vi "Write Interlock.vi"(8 "error in (no error)":errorcluster, 10 "Interlock":bool, 11 "Oven in":refnum<class "Oven.lvclass">) -> (0 "error out":errorcluster, 3 "Oven out":refnum<class "Oven.lvclass">)   [LabVIEW 2018, in "Oven.lvlib" / "Oven.lvclass"]
uses:
  Oven.lvclass
  Oven.lvclass/Oven.ctl
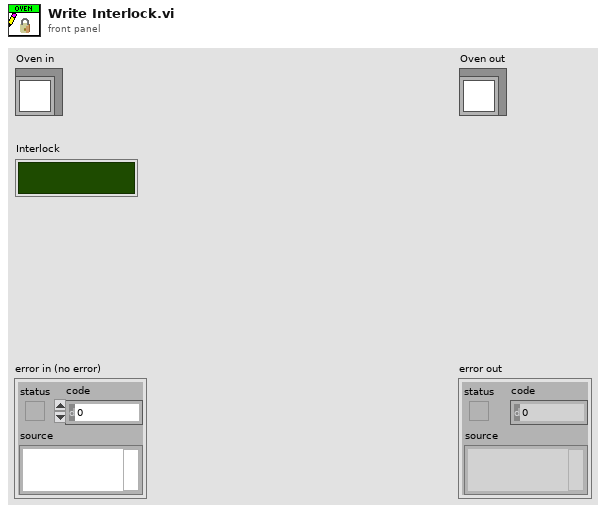
[diagram p1: front panel]
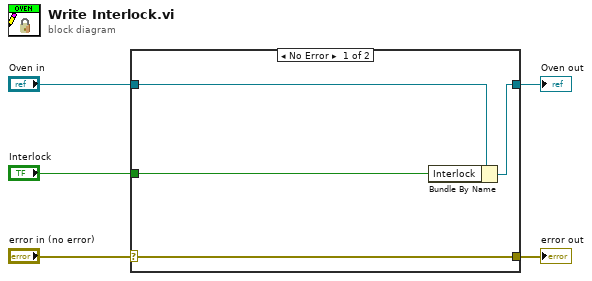
[diagram p0: block diagram]
diagram:
  n1 = case shown="No Error" "error in (no error)" {
    selector: "error in (no error)" -> [w9 w10]
    tunnel: [w9 w10] -> w4
    tunnel: [w7 w11] -> w2
    tunnel: "Oven in" -> [w8 w11]
    tunnel: "Interlock" -> [w6 _]
    frame No Error {
      n2 = Bundle By Name(cluster=w8, "Interlock"=w6) -> (w7:refnum<class "Oven.lvclass">)
    }
    frame Error {
    }
  }
  "error out" <- w4
  "Oven out" <- w2
